vi "Reset wheels.vi"   [LabVIEW 2018]
uses:
  Comulative wheels angles.vi
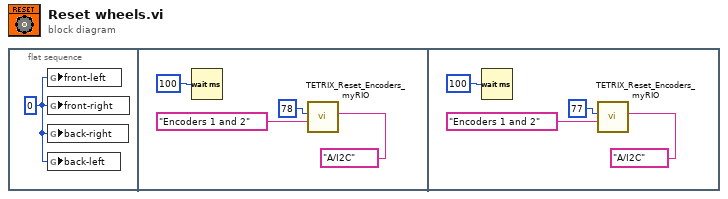
[diagram p0: block diagram]
diagram:
  n1 = flat-sequence {
    frame #0 {
      w1 = 0 ("front-right")
      n2 = global write "Comulative wheels angles.vi" "front-left"(w1) -> ()
      n3 = global write "Comulative wheels angles.vi" "front-right"(w1) -> ()
      n4 = global write "Comulative wheels angles.vi" "back-right"(w1) -> ()
      n5 = global write "Comulative wheels angles.vi" "back-left"(w1) -> ()
    }
    frame #1 {
      n6 = Wait (ms)(milliseconds to wait=u32 100) -> ()  [unwired: 1 out]
      n7 = call <vilib>:"TETRIX_Reset_Encoders_myRIO.vi"("myRIO MXP Port A/B"=tag "A/I2C", "Select Encoder"="Encoders 1 and 2", "Controller ID#  (I2C Address)"=u8 78) -> ()  [unwired: 4 in, 1 out]
    }
    frame #2 {
      n8 = Wait (ms)(milliseconds to wait=u32 100) -> ()  [unwired: 1 out]
      n9 = call <vilib>:"TETRIX_Reset_Encoders_myRIO.vi"("myRIO MXP Port A/B"=tag "A/I2C", "Select Encoder"="Encoders 1 and 2", "Controller ID#  (I2C Address)"=u8 77) -> ()  [unwired: 4 in, 1 out]
    }
  }
